vi "RMS (N Channel).vi"(1 "Array":dbl[][](array[numeric])) -> (0 "Array 2":dbl[](array[numeric]))   [LabVIEW 2017]
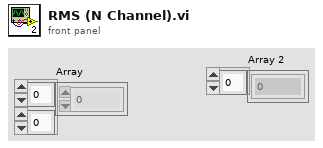
[diagram p1: front panel]
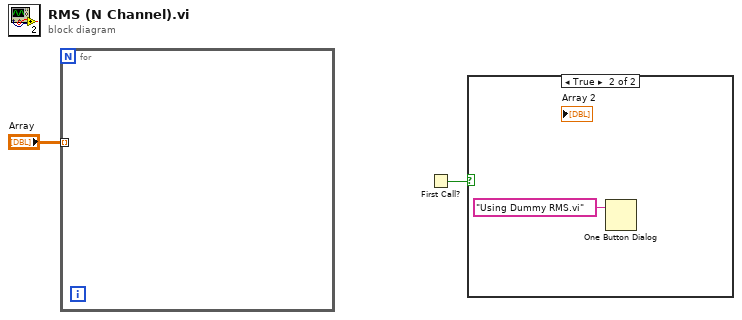
[diagram p0: block diagram]
diagram:
  n1 = for {
    tunnel: "Array" -> [_] mode=indexing
  }
  n2 = First Call?() -> (First Call?: T/F=w2:bool)
  n3 = case shown="True" w2 {
    frame False {
    }
    frame True {
      n4 = One Button Dialog(message="Using Dummy RMS.vi") -> ()  [unwired: 1 in, 1 out]
    }
  }
